vi "VerifyResponse.vi"(8 "error in":errorcluster, 9 "Address #":u8, 10 "Command #":u8, 11 "Data In":T1) -> (0 "error out":errorcluster, 3 "Data out":T1)   [LabVIEW 2020, in "driver_flodx_pressure.lvlib"]
uses:
  <instrlib>/RxnRover/FloDx Pressure Driver/driver_flodx_pressure.lvlib
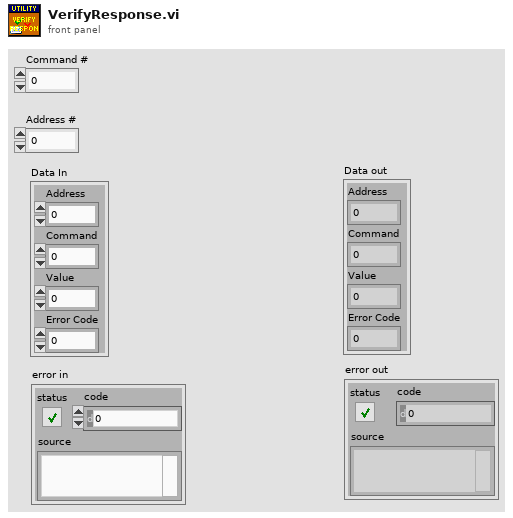
[diagram p1: front panel]
types:
  T1 = cluster{"Address":u32, "Command":u32, "Value":dbl, "Error Code":u32}
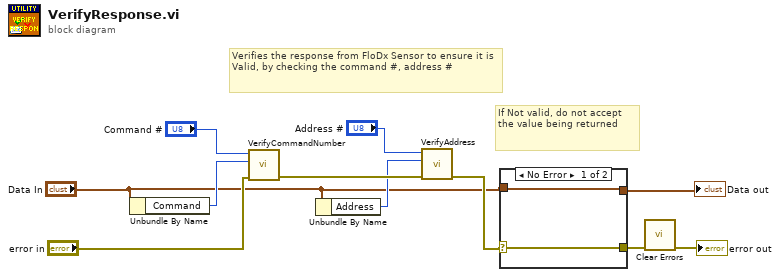
[diagram p0: block diagram]
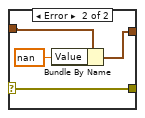
[diagram p2: hidden frame]
diagram:
  # "If Not valid, do not accept the value being returned"
  # "Verifies the response from FloDx Sensor to ensure it is Valid, by checking the command #, address #"
  n1 = Unbundle By Name("Data In") -> ("Command"=w7:u32)
  n2 = call <instrlib>:"VerifyCommandNumber.vi"("error in"="error in", "Command #(From Response)"=w7, "Command #"="Command #") -> ("error out"=w10:errorcluster)  [unwired: 8 in]
  n3 = Unbundle By Name("Data In") -> ("Address"=w6:u32)
  n4 = call <instrlib>:"VerifyAddress.vi"("error in"=w10, "Address(From Response)"=w6, "Address #"="Address #") -> ("error out"=w2:errorcluster)  [unwired: 8 in]
  n5 = case shown="No Error" w2 {
    selector: w2 -> [w13 w17]
    tunnel: [w13 w17] -> w5
    tunnel: [w12 w16] -> w4
    tunnel: "Data In" -> [w12 w14]
    frame No Error {
    }
    frame Error {
      n6 = Bundle By Name(cluster=w14, "Value"=nan) -> (w16:T1)
    }
  }
  "Data out" <- w4
  n7 = call <vilib>:"Clear Errors.vi"("error in (no error)"=w5) -> ("error out"=→"error out":errorcluster)  [unwired: 5 in, 1 out]
